vi "Ramsey Pulse Sequence Generator.vi"(4 "Pulse offset":dbl, 5 "Array":T1(array[cluster]), 6 "MW Delay":dbl, 7 "No. Instructions":i32, 8 "Tau step size":dbl, 9 "Tau max":dbl, 10 "Tau min":dbl, 11 "Rabi Frequency":dbl) -> (2 "Tau":dbl[](array[numeric]), 3 "Pulse Sequence":T1(array[cluster]))   [LabVIEW 2012]
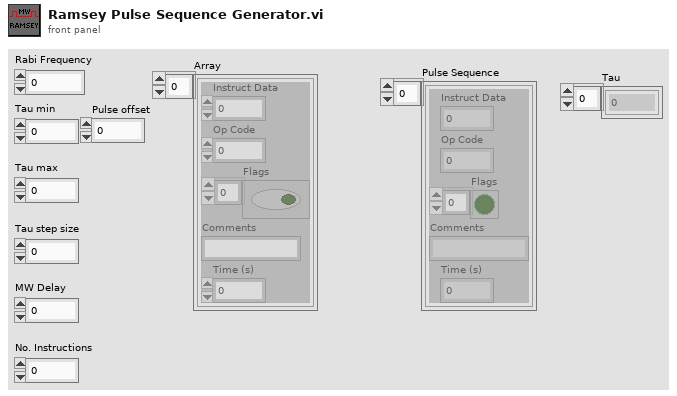
[diagram p1: front panel]
types:
  T1 = cluster{"Instruct Data":i32, "Op Code":i32, "Flags":bool[], "Comments":string, "Time (s)":dbl}[]
  T2 = cluster{"Instruct Data":i32, "Op Code":i32, "Flags":bool[], "Comments":string, "Time (s)":dbl}
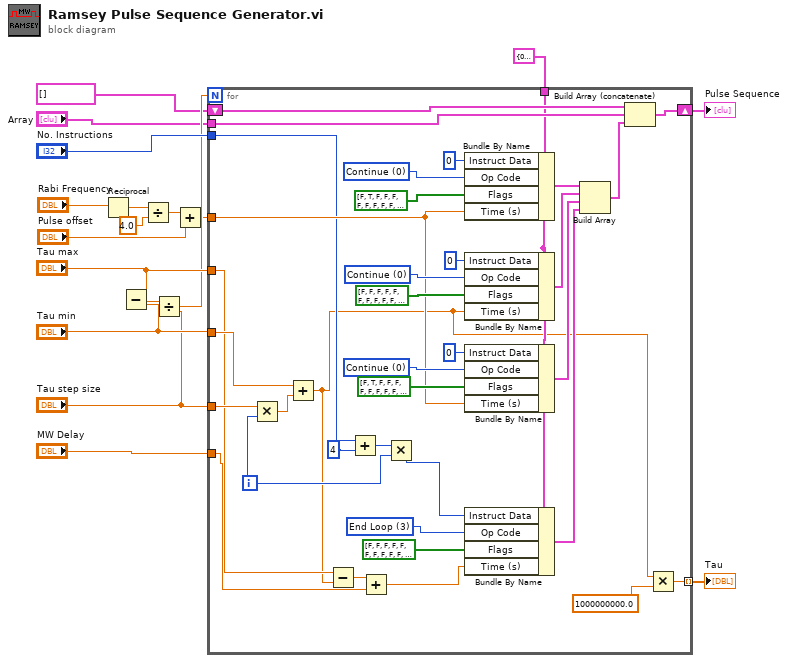
[diagram p0: block diagram]
diagram:
  n1 = Reciprocal(x="Rabi Frequency") -> (1/x=w12:dbl)
  n2 = Subtract(x="Tau max", y="Tau min") -> (x-y=w18:dbl)
  n3 = Divide(x=w12, y=4.0) -> (x/y=w11:dbl)
  n4 = Divide(x=w18, y="Tau step size") -> (x/y=w9:dbl)
  n5 = Add(x=w11, y="Pulse offset") -> (x+y=w2:dbl)
  n6 = for {
    N: w9 -> [_]
    tunnel: "Tau max" -> [w35]
    tunnel: "Tau min" -> [w43]
    tunnel: "Tau step size" -> [w45]
    shift-right: [w52] -> w4
    shift-left: T1 [] -> [w54]
    tunnel: "Array" -> [w53]
    tunnel: "No. Instructions" -> [w26]
    tunnel: T2 {"Instruct Data"=0, "Op Code"=0, "Flags"=[FALSE, FALSE, FALSE, FALSE, FALSE, FALSE, FALSE, FALSE, FALSE, FALSE, FALSE, FALSE, FALSE, FALSE, FALSE, FALSE, FALSE, FALSE, FALSE, FALSE, FALSE, TRUE, TRUE, TRUE], "Comments"="", "Time (s)"=0.01} ("PB Inst 2") -> [w36]
    tunnel: w2 -> [w39]
    tunnel: "MW Delay" -> [w33]
    tunnel: [w19] -> w3 mode=indexing
    i -> [w23]
    w37 = 3 items=["Continue", "Stop", "Loop", "End Loop", "JSR", "RTS", "Branch", "Long Delay", "Wait"] ("Op Code")
    w41 = 0 items=["Continue", "Stop", "Loop", "End Loop", "JSR", "RTS", "Branch", "Long Delay", "Wait"] ("Op Code")
    w47 = 0 items=["Continue", "Stop", "Loop", "End Loop", "JSR", "RTS", "Branch", "Long Delay", "Wait"] ("Op Code")
    w50 = 0 items=["Continue", "Stop", "Loop", "End Loop", "JSR", "RTS", "Branch", "Long Delay", "Wait"] ("Op Code")
    n7 = Multiply(x=w45, y=w23) -> (x*y=w44:dbl)
    n8 = Add(x=w43, y=w44) -> (x+y=w20:dbl)
    n9 = Subtract(x=w35, y=w20) -> (x-y=w34:dbl)
    n10 = Add(x=w26, y=4) -> (x+y=w24:i32)
    n11 = Add(x=w34, y=w33) -> (x+y=w32:dbl)
    n12 = Multiply(x=w24, y=w23) -> (x*y=w22:i32)
    n13 = Bundle By Name(cluster=w36, "Instruct Data"=0, "Op Code"=w50, "Flags"=bool[] [FALSE, TRUE, FALSE, FALSE, FALSE, FALSE, FALSE, FALSE, FALSE, FALSE, FALSE, FALSE, FALSE, FALSE, FALSE, FALSE, FALSE, FALSE, FALSE, FALSE, FALSE, TRUE, TRUE, TRUE], "Time (s)"=w39) -> (w31:T2)
    n14 = Bundle By Name(cluster=w36, "Instruct Data"=0, "Op Code"=w47, "Flags"=bool[] [FALSE, FALSE, FALSE, FALSE, FALSE, FALSE, FALSE, FALSE, FALSE, FALSE, FALSE, FALSE, FALSE, FALSE, FALSE, FALSE, FALSE, FALSE, FALSE, FALSE, FALSE, TRUE, TRUE, TRUE], "Time (s)"=w20) -> (w28:T2)
    n15 = Bundle By Name(cluster=w36, "Instruct Data"=0, "Op Code"=w41, "Flags"=bool[] [FALSE, TRUE, FALSE, FALSE, FALSE, FALSE, FALSE, FALSE, FALSE, FALSE, FALSE, FALSE, FALSE, FALSE, FALSE, FALSE, FALSE, FALSE, FALSE, FALSE, FALSE, TRUE, TRUE, TRUE], "Time (s)"=w39) -> (w29:T2)
    n16 = Bundle By Name(cluster=w36, "Instruct Data"=w22, "Op Code"=w37, "Flags"=bool[] [FALSE, FALSE, FALSE, FALSE, FALSE, FALSE, FALSE, FALSE, FALSE, FALSE, FALSE, FALSE, FALSE, FALSE, FALSE, FALSE, FALSE, FALSE, FALSE, FALSE, FALSE, TRUE, TRUE, TRUE], "Time (s)"=w32) -> (w30:T2)
    n17 = Build Array(w31, w28, w29, w30) -> (w27:T1)
    n18 = Build Array (concatenate)(w54, w53, w27) -> (w52:T1)
    n19 = Multiply(x=w20, y=1000000000.0) -> (x*y=w19:dbl)
  }
  "Pulse Sequence" <- w4
  "Tau" <- w3
